vi "Get Icon from Generic.vi"(8 "error in":errorcluster, 11 "GObj Ref in":refnum<vi>) -> (0 "error out":errorcluster, 1 "Found":bool, 2 "Icon out":refnum<class "Icon.lvclass">, 3 "GObj Ref out":refnum<vi>)   [LabVIEW 2024, in "XNode Support.lvlib"]
doc: "Read LabVIEW Icon Data from a VI."
uses:
  XNode Support.lvlib
  <vilib>/LabVIEW Icon API/lv_icon/Classes/Icon/Icon.lvclass
  <vilib>/LabVIEW Icon API/lv_icon/lv_icon.lvlib
  <vilib>/LabVIEW Icon API/lv_icon/Controls/Alignment.ctl
  <vilib>/LabVIEW Icon API/lv_icon/Controls/Font.ctl
  <vilib>/LabVIEW Icon API/lv_icon/Controls/BodyText.ctl
  <vilib>/LabVIEW Icon API/LabVIEW Icon API.lvlib
  <vilib>/picture/picture.llb/imagedata.ctl
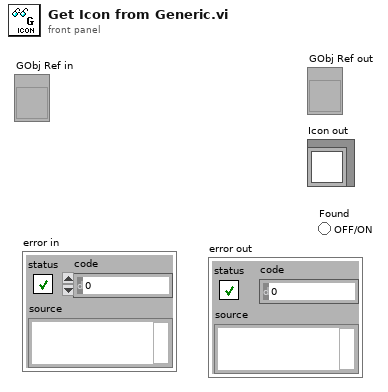
[diagram p1: front panel]
types:
  T1 = typedef "imagedata.ctl" = cluster{"image type":i32, "image depth":i32, "image":u8[], "mask":u8[], "colors":u32[], "Rectangle":cluster{"left":i16, "top":i16, "right":i16, "bottom":i16}}
  T2 = typedef "BodyText.ctl" = cluster{"Line 1 text":string, "Line 2 text":string, "Line 3 text":string, "Line 4 text":string, "Line 1 color":u32, "Line 2 color":u32, "Line 3 color":u32, "Line 4 color":u32, "Body Text Spec":cluster{"Font":T3, "Alignment":T4, "Size":u8}, "Center text vertically":bool, "Capitalize Text":bool}
  T3 = typedef "Font.ctl" = string
  T4 = typedef "Alignment.ctl" = u16
  T5 = typedef "LabVIEW Icon Stored Information.ctl" = cluster{"Text Visible?":bool, "Text Opacity":u8, "Templ Visible?":bool, "Templ Opacity":u8, "Relative Path from 1 to 2":path, "Image":picture, "All User Layers":refnum<class "Layer.lvclass">[], "Body Text":T2}
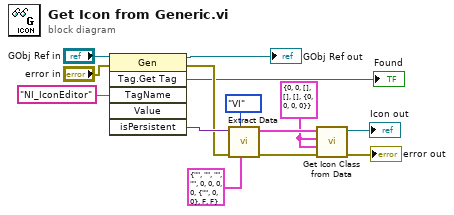
[diagram p0: block diagram]
diagram:
  w2 = T1 {"image type"=0, "image depth"=0, "image"=[], "mask"=[], "colors"=[], "Rectangle"={"left"=0, "top"=0, "right"=0, "bottom"=0}} ("Color Icon")
  n1 = invoke class="Gen" method="Tag.Get Tag"(reference="GObj Ref in", error in="error in", "TagName"="NI_IconEditor" ("Tag Name")) -> (reference out=→"GObj Ref out":refnum<vi>, error out=w9:errorcluster, "GetTag"=→"Found":bool, "isPersistent"=w12:variant)  [unwired: 3 in, 2 out]
  n2 = call <vilib>:"Extract Data.vi"("Default body text"=T2 {"Line 1 text"="", "Line 2 text"="", "Line 3 text"="", "Line 4 text"="", "Line 1 color"=0, "Line 2 color"=0, "Line 3 color"=0, "Line 4 color"=0, "Body Text Spec"={"Font"="", "Alignment"=0, "Size"=0}, "Center text vertically"=FALSE, "Capitalize Text"=FALSE}, "Type"=enum16{"VI", "Library"}."VI", "error in"=w9, "Value"=w12) -> ("error out"=w3:errorcluster, "Data"=w6:T5)  [unwired: 1 in, 5 out]
  n3 = call <vilib>:"Get Icon Class from Data.vi"("error in (no error)"=w3, "BW Icon"=w2, "Color Icon"=w2, "Icon Data"=w6) -> ("error out"=→"error out":errorcluster, "Icon out"=→"Icon out":refnum<class "Icon.lvclass">)  [unwired: 6 in]
